vi "写入PN.vi"(0 "产品名":string, 5 "型号":string, 7 "版本号":string, 9 "产品料号":string, 11 "流水号":string, 12 "error in":errorcluster) -> (4 "return":i32, 13 "error out":errorcluster)   [LabVIEW 2016]
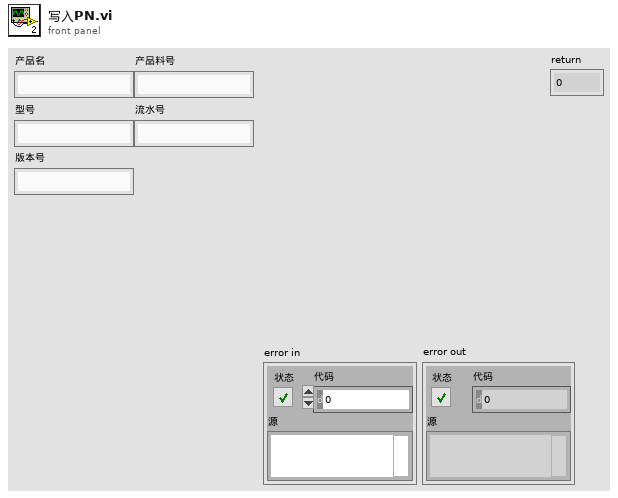
[diagram p1: front panel]
types:
  T1 = cluster{"byCmdType":u8, "bySubCmd":u8, "byPara":u8, "byAddr_h":u8, "byAddr_l":u8, "byAddr_ll":u8, "byLen_h":u8, "byLen_l":u8}
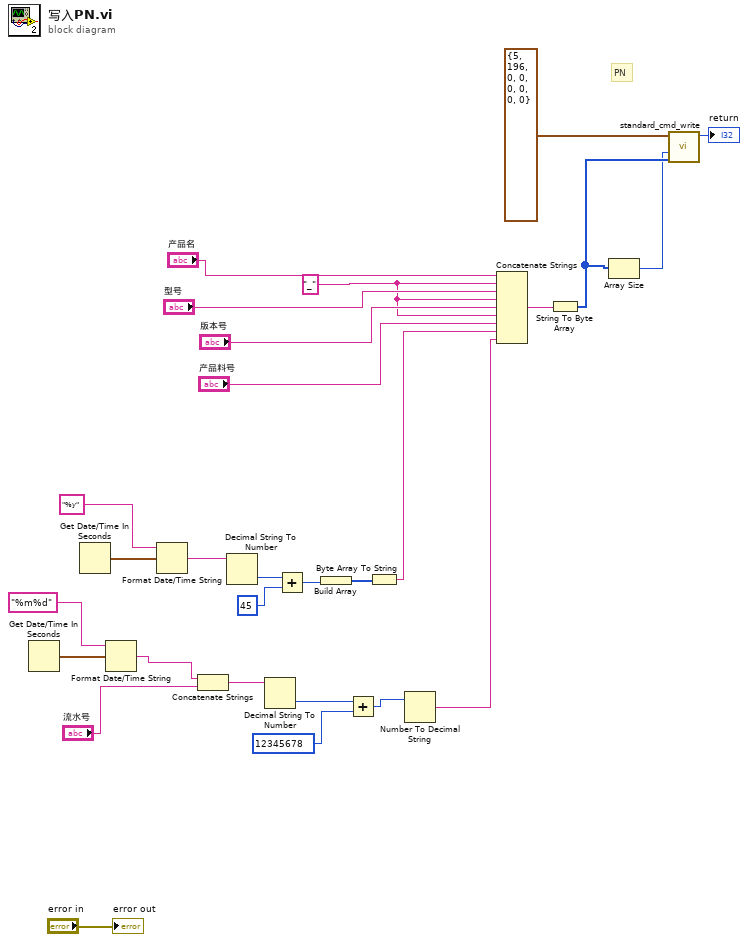
[diagram p0: block diagram]
diagram:
  w13 = "_"
  # "PN"
  n1 = Get Date/Time In Seconds() -> (seconds since 1Jan1904=w24:timestamp)
  n2 = Get Date/Time In Seconds() -> (seconds since 1Jan1904=w27:timestamp)
  n3 = Format Date/Time String(time format string (%c)="%m%d", seconds (now)=w24) -> (date/time string=w7:string)  [unwired: 1 in]
  n4 = Format Date/Time String(time format string (%c)="%y", seconds (now)=w27) -> (date/time string=w23:string)  [unwired: 1 in]
  n5 = Concatenate Strings(w7, "流水号") -> (w5:string)
  n6 = Decimal String To Number(string=w23) -> (number=w22:i32)  [unwired: 2 in, 1 out]
  n7 = Decimal String To Number(string=w5) -> (number=w4:i32)  [unwired: 2 in, 1 out]
  n8 = Add(x=w22, y=45) -> (x+y=w20:i32)
  n9 = Build Array(w20) -> (w19:i32[])
  n10 = Add(x=w4, y=12345678) -> (x+y=w2:i32)
  n11 = Byte Array To String(unsigned byte array=w19) -> (string=w14:string)
  n12 = Number To Decimal String(number=w2) -> (decimal integer string=w1:string)  [unwired: 1 in]
  n13 = Concatenate Strings("产品名", w13, "型号", w13, "版本号", w13, "产品料号", w14, w1) -> (w12:string)
  n14 = String To Byte Array(string=w12) -> (unsigned byte array=w11:u8[])
  n15 = Array Size(array=w11) -> (size(s)=w10:i32)
  n16 = call "standard_cmd_write.vi"("data"=w11, "dwLen"=w10, "cmd_std_header_t"=T1 {"byCmdType"=5, "bySubCmd"=196, "byPara"=0, "byAddr_h"=0, "byAddr_l"=0, "byAddr_ll"=0, "byLen_h"=0, "byLen_l"=0}) -> ("return"=→"return":i32)  [unwired: 7 in, 1 out]
  "error out" <- "error in"
